vi "rethinkdb_json_tokenize.vi"(8 "error in (no error)":errorcluster, 11 "json":string) -> (0 "error out":errorcluster, 1 "invalid?":bool, 2 "args":string[](array[string]), 3 "tokens":T1[](array[typedef]))   [LabVIEW 2017]
uses:
  rethinkdb_json_token.ctl
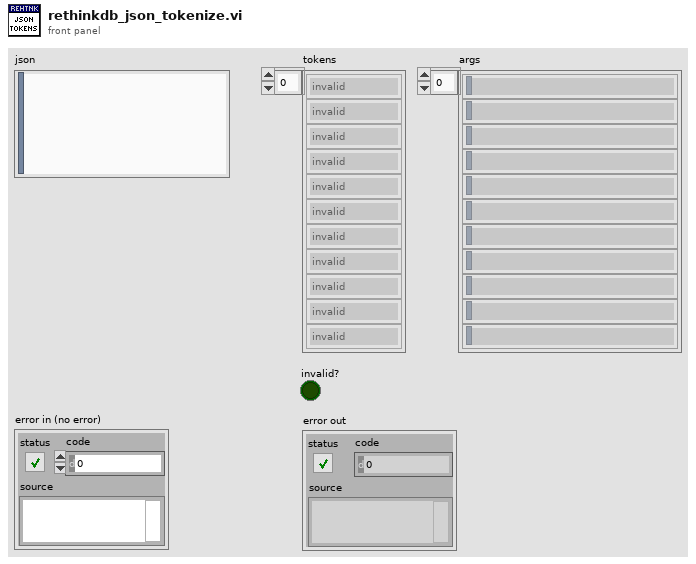
[diagram p1: front panel]
types:
  T1 = typedef "rethinkdb_json_token.ctl" = enum8{"invalid", "null", "boolean", "decimal", "float", "string", "key", "comma", "object_start", "object_end", "array_start", "array_end", "end"}
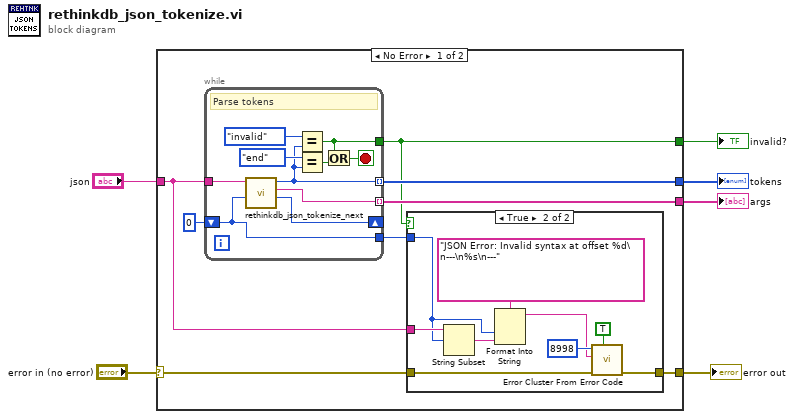
[diagram p0: block diagram]
diagram:
  n1 = case shown="No Error" "error in (no error)" {
    selector: "error in (no error)" -> [w11 w35]
    tunnel: "json" -> [w9 _]
    tunnel: [w13 _] -> w5
    tunnel: [w12 _] -> w4
    tunnel: [w7 _] -> w3
    tunnel: [w10 w35] -> w1
    frame No Error {
      n2 = while {
        tunnel: w9 -> [w34]
        shift-right: [w33] -> _
        shift-left: 0 ("offset past token") -> [w25]
        tunnel: [w28] -> w13 mode=indexing
        tunnel: [w27] -> w12 mode=indexing
        tunnel: [w26] -> w7
        tunnel: [w25] -> w8
        stop <- w29 stop-if-true
        # "Parse tokens"
        n3 = call "rethinkdb_json_tokenize_next.vi"("offset (0)"=w25, "json"=w34) -> ("offset past token"=w33:i32, "arg"=w27:string, "token"=w28:T1)  [unwired: 7 in]
        n4 = Equal?(x=rethinkdb_json_token."invalid", y=w28) -> (x = y?=w26:bool)
        n5 = Equal?(x=rethinkdb_json_token."end", y=w28) -> (x = y?=w30:bool)
        n6 = Or(x=w26, y=w30) -> (x .or. y?=w29:bool)
      }
      n7 = case shown="True" w7 {
        tunnel: w11 -> [w15 w24]
        tunnel: [w15 w23] -> w10
        tunnel: w9 -> [_ w20]
        tunnel: w8 -> [_ w17]
        frame False {
        }
        frame True {
          n8 = String Subset(string=w20, offset (0)=w17) -> (substring=w19:string)  [unwired: 1 in]
          n9 = Format Into String(format string="JSON Error: Invalid syntax at offset %d\n---\n%s\n---" ("error message (\"\")"), w17, w19) -> (resulting string=w16:string)  [unwired: 2 in, 1 out]
          n10 = call <vilib>:"Error Cluster From Error Code.vi"("show call chain? (False)"=TRUE, "error in (no error)"=w24, "error message (\"\")"=w16, "error code (0)"=8998) -> ("error out"=w23:errorcluster)  [unwired: 5 in]
        }
      }
    }
    frame Error {
    }
  }
  "tokens" <- w5
  "args" <- w4
  "invalid?" <- w3
  "error out" <- w1
